vi "Reset.vi"(8 "error in (no error)":errorcluster, 11 "VISA resource name":refnum<visa-resource-name>) -> (0 "error out":errorcluster, 3 "VISA resource name out":refnum<visa-resource-name>)   [LabVIEW 2020, in "Template - Register.lvlib"]
doc: "Resets the instrument, and then sets the instrument into the default state."
uses:
  <instrlib>/_Template - Register/Template - Register.lvlib
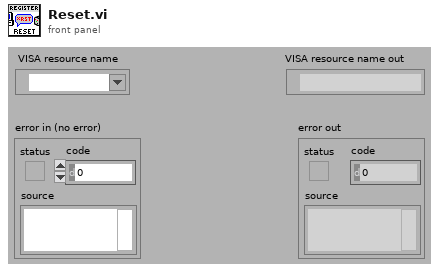
[diagram p1: front panel]
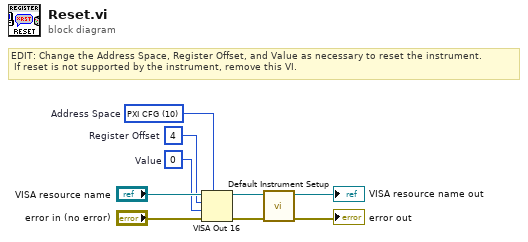
[diagram p0: block diagram]
diagram:
  w1 = u16 0  # Value
  w2 = u32 4  # Register Offset
  w3 = u16 10 items=["A16"=1, "A24"=2, "A32"=3, "PXI CFG"=10, "PXI BAR0"=11, "PXI BAR1"=12, "PXI BAR2"=13, "PXI BAR3"=14, "PXI BAR4"=15, "PXI BAR5"=16]  # Address Space
  # "EDIT: Change the Address Space, Register Offset, and Value as necessary to reset the instrument.\n If reset is not supported by the instrument, remove this VI."
  n1 = VISA Out 16(7:w3, 8:"error in (no error)", 9:w1, 10:w2, 11:"VISA resource name") -> (0:w4:errorcluster, 3:w6:refnum<visa-resource-name>)
  n2 = call <instrlib>:"Default Instrument Setup.vi"("error in (no error)"=w4, "VISA resource name"=w6) -> ("error out"=→"error out":errorcluster, "VISA resource name out"=→"VISA resource name out":refnum<visa-resource-name>)  [unwired: 8 in]
